vi "BT Example 4 - Sequence to Modularise Tree.vi"() -> ()   [LabVIEW 2021]
uses:
  Support/Nodes/abs_Node/Status.ctl
  Blackboard/Blackboard.lvclass
  Support/Nodes/Decorators/Repeater/Support/Finish On - Type.ctl
  System/bt_System.lvclass
  Blackboard/Blackboard.lvclass/Blackboard.ctl
  Support/Nodes/Leaves/abs_Type Leaf/abs_Type Leaf.lvclass/abs_Type Leaf.ctl
  Blackboard/Get Value Type/Get I32.vi
  Blackboard/Get Value Type/Get Boolean.vi
  <vilib>/TSA/Abstract Data Classes/Abs_Types/I32 Integer/Static Read.vi
  <vilib>/TSA/Abstract Data Classes/Abs_Types/Boolean/Static Read.vi
  Blackboard/Support/Index Group.vi
  Blackboard/Support/Index Tags.vi
  Support/Nodes/Leaves/abs_Type Leaf/Properties/Write Value Class.vi
  <vilib>/TSA/Omni-Bus/Local Bus/Support/I32/Local Bus_I32.lvclass
  C:/Program Files (x86)/National Instruments/LabVIEW 2021/vi.lib/TSA/Abstract Data Classes/Abs_Types/Value/Abs_Value.lvclass
  <vilib>/TSA/Abstract Data Classes/Abs_Types/I32 Integer/Abs_I32 Integer.lvclass
  <vilib>/TSA/Omni-Bus/Local Bus/Support/Bool/Local Bus_Boolean.lvclass
  <vilib>/TSA/Abstract Data Classes/Abs_Types/Boolean/Abs_Boolean.lvclass
  C:/Program Files (x86)/National Instruments/LabVIEW 2021/vi.lib/TSA/Abstract Data Classes/Abs_Types/Type/Abs_Type.lvclass
  Support/Nodes/Leaves/Test Boolean/Test Abs_Boolean.lvclass
  C:/Users/Tim/Documents/GitHub/LV_Behaviour_Tree/Source/Support/Nodes/abs_Node/bt_Node.lvclass
  C:/Users/Tim/Documents/GitHub/LV_Behaviour_Tree/Source/Support/Nodes/Leaves/abs_Type Leaf/abs_Type Leaf.lvclass
  <vilib>/TSA/Abstract Data Classes/Constants/Support/Bool/Bool.vi
  <vilib>/TSA/Omni-Bus/Local Bus/Support/Initialise DVR's.vi
  <vilib>/TSA/Abstract Data Classes/Functions/Math/Support/Increment/I32/Method.vi
  <vilib>/TSA/Abstract Data Classes/Functions/Compare/Support/Less/I32/Method_Const.vi
  <vilib>/TSA/Abstract Data Classes/Abs_Types/Value/Abs_Value.lvclass
  <vilib>/TSA/Abstract Data Classes/Abs_Types/Type/Abs_Type.lvclass
  <vilib>/TSA/Omni-Bus/Local Bus/Support/DBL/Local Bus_DBL.lvclass
  <vilib>/TSA/Omni-Bus/Local Bus/Support/SGL/Local Bus_SGL.lvclass
  <vilib>/TSA/Omni-Bus/Local Bus/Support/EXT/Local Bus_EXT.lvclass
  <vilib>/TSA/Omni-Bus/Local Bus/Support/STR/Local Bus_String.lvclass
  <vilib>/TSA/Omni-Bus/Local Bus/Support/Variant/Local Bus_Variant.lvclass
  <vilib>/TSA/Omni-Bus/Local Bus/Support/WFM/Local Bus_Waveform.lvclass
  <vilib>/TSA/Omni-Bus/Local Bus/Support/Time/Local Bus_Time.lvclass
  <vilib>/TSA/Omni-Bus/Local Bus/Support/U8/Local Bus_U8.lvclass
  <vilib>/TSA/Omni-Bus/Local Bus/Support/U16/Local Bus_U16.lvclass
  <vilib>/TSA/Omni-Bus/Local Bus/Support/U32/Local Bus_U32.lvclass
  <vilib>/TSA/Omni-Bus/Local Bus/Support/U64/Local Bus_U64.lvclass
  <vilib>/TSA/Omni-Bus/Local Bus/Support/I8/Local Bus_I8.lvclass
  <vilib>/TSA/Omni-Bus/Local Bus/Support/I16/Local Bus_I16.lvclass
  <vilib>/TSA/Omni-Bus/Local Bus/Support/I64/Local Bus_I64.lvclass
  <vilib>/TSA/Omni-Bus/Local Bus/Support/CSGL/Local Bus_CSGL.lvclass
  <vilib>/TSA/Omni-Bus/Local Bus/Support/CDBL/Local Bus_CDBL.lvclass
  <vilib>/TSA/Omni-Bus/Local Bus/Support/CEXT/Local Bus_CEXT.lvclass
  BT.lvlib
  Support/Nodes/Decorators/Repeater/bt_Repeater.lvclass
  <vilib>/TSA/Abstract Data Classes/Constants/Support/Bool/Const_Bool.lvclass
  Support/Nodes/abs_Node/bt_Node.lvclass
  <vilib>/TSA/Abstract Data Classes/Functions/Compare/Support/Less/I32/Less_I32.lvclass
  <vilib>/TSA/Abstract Data Classes/Functions/Math/Support/Increment/I32/Increment_I32.lvclass
panel:
  out "Count":i32
  out "Status":T1
  out "Indicators":bool[](array[boolean])
  in  "stop":bool
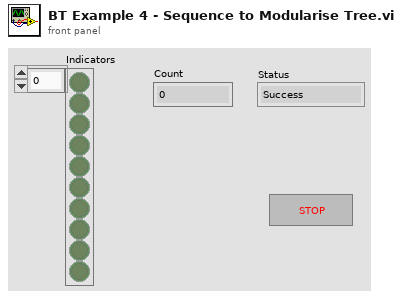
[diagram p1: front panel]
types:
  T1 = typedef "BT.lvlib/bt_Node.lvclass/Status.ctl" = enum16{"Success", "Failure", "Running"}
  T2 = typedef "BT.lvlib/bt_Repeater.lvclass/Finish On - Type.ctl" = enum16{"Success", "Failure", "Never"}
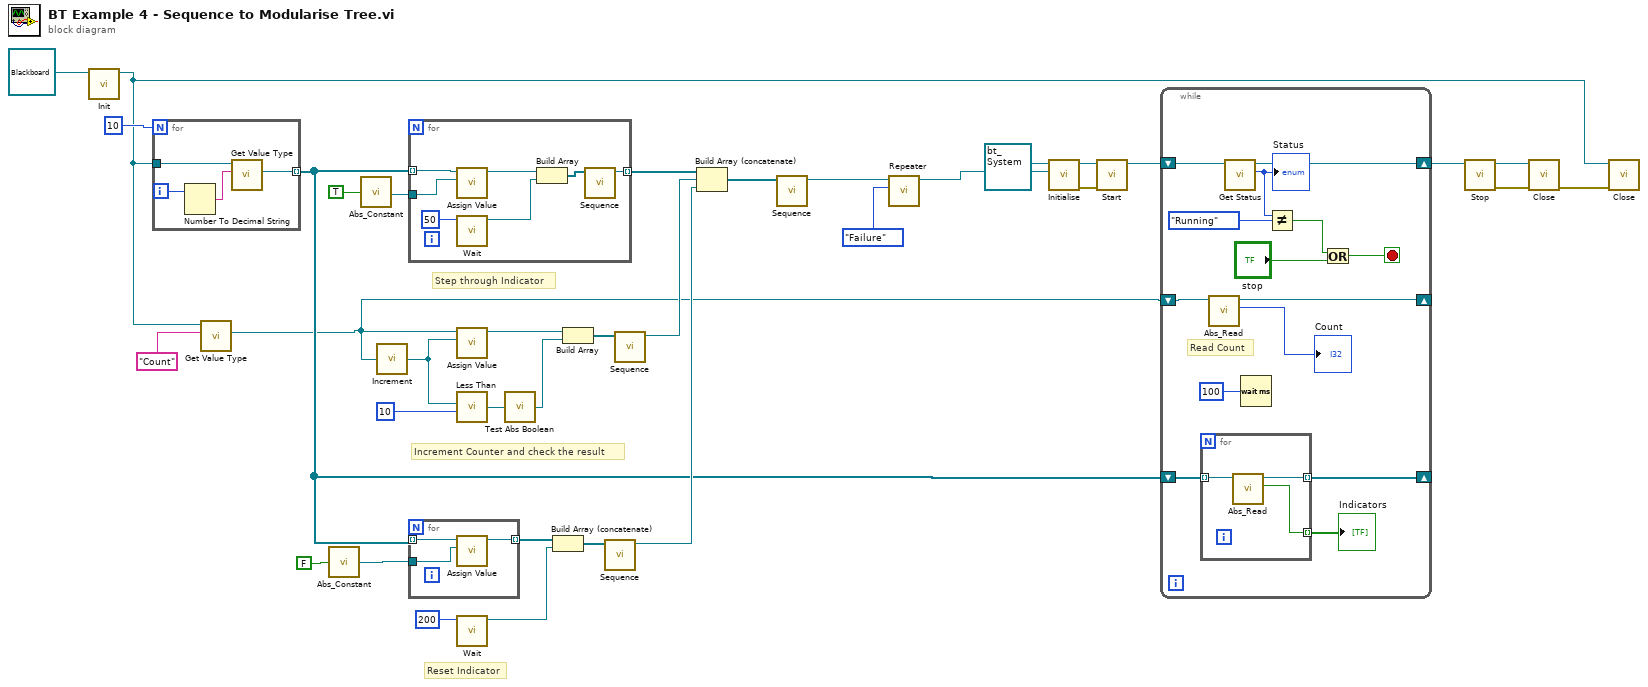
[diagram p0: block diagram]
diagram:
  # "Step through Indicator"
  # "Increment Counter and check the result"
  # "Reset Indicator"
  n1 = call-dynamic "Init.vi"("bt_Blackboard in"=refnum<class "Blackboard.lvclass"> refnum) -> ("bt_Blackboard out"=w3:refnum<class "Blackboard.lvclass">)  [unwired: 9 in, 1 out]
  n2 = for {
    N: 10 -> [_]
    tunnel: w3 -> [w39]
    tunnel: [w38] -> w2 mode=indexing
    i -> [w36]
    n3 = Number To Decimal String(number=w36) -> (decimal integer string=w37:string)  [unwired: 1 in]
    n4 = call-poly "Get Value Type.vi"("Tag"=w37, "Blackboard in"=w39) -> ("Value"=w38:refnum<class "Abs_Boolean.lvclass">)  [unwired: 6 in, 3 out]
  }
  n5 = call-poly "Get Value Type.vi"("Tag"="Count", "Blackboard in"=w3) -> ("Value"=w1:refnum<class "Abs_I32 Integer.lvclass">)  [unwired: 6 in, 3 out]
  n6 = call-poly <vilib>:"Abs_Constant.vi"("Boolean"=FALSE) -> ("Abs_Boolean.lvclass"=w20:refnum<class "Abs_Boolean.lvclass">)  [unwired: 4 in]
  n7 = call-poly <vilib>:"Abs_Constant.vi"("Boolean"=TRUE) -> ("Abs_Boolean.lvclass"=w21:refnum<class "Abs_Boolean.lvclass">)  [unwired: 4 in]
  n8 = call-poly <vilib>:"Increment.vi"("Value"=w1) -> ("Result"=w15:refnum<class "Abs_I32 Integer.lvclass">)  [unwired: 4 in]
  n9 = for {
    tunnel: w21 -> [w46]
    tunnel: w2 -> [w41] mode=indexing
    tunnel: [w40] -> w13 mode=indexing
    n10 = call "Assign Value.vi"("Assigned Value"=w46, "Value"=w41) -> ("Node Out"=w45:refnum<class "bt_Node.lvclass">)  [unwired: 9 in]
    n11 = call "Wait.vi"("Time (ms)"=u32 50) -> ("Node Out"=w44:refnum<class "bt_Node.lvclass">)  [unwired: 10 in]
    n12 = Build Array(w45, w44) -> (w43:refnum<class "bt_Node.lvclass">[])
    n13 = call "Sequence.vi"("Nodes"=w43) -> ("Node"=w40:refnum<class "bt_Node.lvclass">)  [unwired: 10 in]
  }
  n14 = for {
    tunnel: w20 -> [w49]
    tunnel: w2 -> [w48] mode=indexing
    tunnel: [w47] -> w12 mode=indexing
    n15 = call "Assign Value.vi"("Assigned Value"=w49, "Value"=w48) -> ("Node Out"=w47:refnum<class "bt_Node.lvclass">)  [unwired: 9 in]
  }
  n16 = call "Assign Value.vi"("Assigned Value"=w15, "Value"=w1) -> ("Node Out"=w8:refnum<class "bt_Node.lvclass">)  [unwired: 9 in]
  n17 = call-poly <vilib>:"Less Than.vi"("Value"=10, "Value A"=w15) -> ("Result"=w16:refnum<class "Abs_Boolean.lvclass">)  [unwired: 4 in]
  n18 = call "Wait.vi"("Time (ms)"=u32 200) -> ("Node Out"=w11:refnum<class "bt_Node.lvclass">)  [unwired: 10 in]
  n19 = call "Test Abs Boolean.vi"("Abs_Boolean.lvclass"=w16) -> ("abs_Node"=w7:refnum<class "bt_Node.lvclass">)  [unwired: 4 in]
  n20 = Build Array (concatenate)(w12, w11) -> (w10:refnum<class "bt_Node.lvclass">[])
  n21 = Build Array(w8, w7) -> (w9:refnum<class "bt_Node.lvclass">[])
  n22 = call "Sequence.vi"("Nodes"=w10) -> ("Node"=w5:refnum<class "bt_Node.lvclass">)  [unwired: 10 in]
  n23 = call "Sequence.vi"("Nodes"=w9) -> ("Node"=w6:refnum<class "bt_Node.lvclass">)  [unwired: 10 in]
  n24 = Build Array (concatenate)(w13, w6, w5) -> (w23:refnum<class "bt_Node.lvclass">[])
  n25 = call "Sequence.vi"("Nodes"=w23) -> ("Node"=w24:refnum<class "bt_Node.lvclass">)  [unwired: 10 in]
  n26 = call "Repeater.vi"("Finish On"=Finish_On_-_Type."Failure", "Node In"=w24) -> ("Node Out"=w26:refnum<class "bt_Node.lvclass">)  [unwired: 9 in]
  n27 = call "Initialise.vi"("Behaviour Tree"=w26, "bt_System in"=refnum<class "bt_System.lvclass"> refnum) -> ("error out"=w27:errorcluster, "bt_System out"=w28:refnum<class "bt_System.lvclass">)  [unwired: 8 in]
  n28 = call "Start.vi"("error in (no error)"=w27, "bt_System in"=w28) -> ("bt_System out"=w35:refnum<class "bt_System.lvclass">)  [unwired: 8 in, 1 out]
  n29 = while {
    shift-right: [w58] -> w34
    shift-left: w35 -> [w59]
    shift-right: [w62] -> _
    shift-left: w2 -> [w63]
    shift-right: [w50] -> _
    shift-left: w1 -> [w51]
    stop <- w56 stop-if-true
    # "Read Count"
    n30 = for {
      tunnel: w63 -> [w66] mode=indexing
      tunnel: [w65] -> w62 mode=indexing
      tunnel: [w64] -> w61 mode=indexing
      n31 = call-poly <vilib>:"Abs_Read.vi"("Abs_Boolean in"=w66) -> ("Boolean"=w64:bool, "Abs_Boolean out"=w65:refnum<class "Abs_Boolean.lvclass">)  [unwired: 8 in, 1 out]
    }
    "Indicators" <- w61
    n32 = call-poly <vilib>:"Abs_Read.vi"("Abs_I32 Integer in"=w51) -> ("Value"=→"Count":i32, "Abs_I32 Integer out"=w50:refnum<class "Abs_I32 Integer.lvclass">)  [unwired: 8 in, 1 out]
    n33 = call "Get Status.vi"("bt_System in"=w59) -> ("Status"=w55:T1, "bt_System out"=w58:refnum<class "bt_System.lvclass">)  [unwired: 8 in, 1 out]
    "Status" <- w55
    n34 = Wait (ms)(milliseconds to wait=u32 100) -> ()  [unwired: 1 out]
    n35 = Not Equal?(x=w55, y=Status."Running") -> (x != y?=w53:bool)
    n36 = Or(x=w53, y="stop") -> (x .or. y?=w56:bool)
  }
  n37 = call "Stop.vi"("bt_System in"=w34) -> ("error out"=w29:errorcluster, "bt_System out"=w30:refnum<class "bt_System.lvclass">)  [unwired: 9 in]
  n38 = call-dynamic "Close.vi"("error in (no error)"=w29, "bt_System in"=w30) -> ("error out"=w33:errorcluster)  [unwired: 8 in, 1 out]
  n39 = call-dynamic "Close.vi"("error in (no error)"=w33, "bt_Blackboard in"=w3) -> ()  [unwired: 8 in, 2 out]
